vi "rm.server.visualize.get resource entries.vi"(7 "show unmapped?":bool, 8 "error in (no error)":errorcluster, 11 "Item Ref in":T2 format="%.0x") -> (0 "error out":errorcluster, 2 "resource entries":T1[](array[typedef]) {"FPGA CD Ref" format="%.0x"; "reserver" format="%.0x"}, 3 "Item Ref out":T2 format="%.0x")   [LabVIEW 2016, in "RM.Server.lvlib"]
uses:
  RM.Server.lvlib
  <vilib>/NI Veristand/Custom Device API/Custom Device Item Ref.ctl
  viz_entry.ctl
  FPGA-Addon/Source/Shared/FG Action.ctl
  FPGA-Addon/Source/Shared/Constants.vi
  <vilib>/NI Veristand/Custom Device API/Get Item Property (Variant).vi
  <vilib>/NI Veristand/Custom Device API/NI VeriStand - Set Item Property.vi
  <vilib>/NI Veristand/Custom Device API/Set Item Property (Variant).vi
  <vilib>/NI Veristand/Custom Device API/Get Item Property (Dependent Node Pointer).vi
  <vilib>/NI Veristand/Custom Device API/Get Item Property (String).vi
  <vilib>/NI VeriStand/Custom Device API/Custom Device API.lvlib
  FPGA-Addon/Source/Shared/FPGA Addon Shared.lvlib
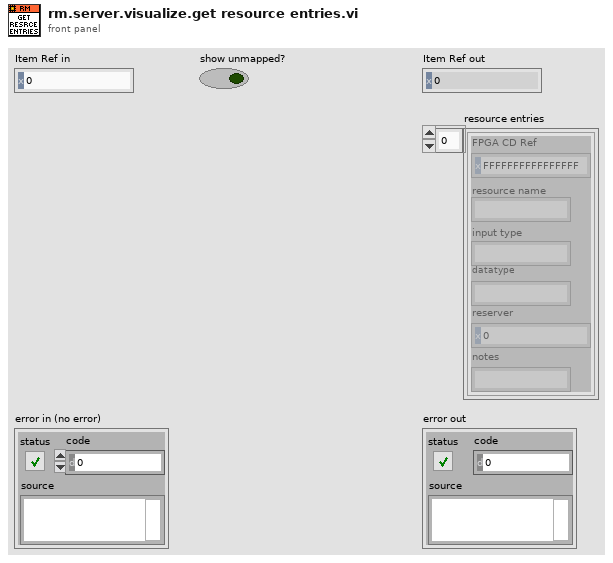
[diagram p1: front panel]
types:
  T1 = typedef "RM.Server.lvlib/viz_entry.ctl" = cluster{"FPGA CD Ref":T2, "resource name":string, "input type":string, "datatype":string, "reserver":T2, "notes":string}
  T2 = typedef "Custom Device API.lvlib/Custom Device Item Ref.ctl" = u64
  T3 = typedef "FPGA Addon Shared.lvlib/FG Action.ctl" = enum8{"GET", "SET"}
  T4 = typedef "Custom Device API.lvlib/Custom Device Item Info.ctl" = cluster{"Name":string, "Is Channel":bool, "GUID":string, "Is Waveform":bool}
  T5 = typedef "FPGA Addon Shared.lvlib/Register Information.ctl" = cluster{"Name":string, "Data Type":T6, "Default Value":variant}
  T6 = typedef "FPGA Addon Shared.lvlib/Data Type.ctl" = enum8{"<Null>", "I8", "I16", "I32", "I64", "U8", "U16", "U32", "U64", "SGL", "Boolean", "Analog PWM In Settings", "Analog PWM In", "Digital PWM In Settings", "Digital PWM In", "Digital PWM Out", "Sine Out", "FXP+/-24.5", "FXP+/-16.5", "FXP+/-32.8", "FXP+/-64.32", "FXP+/-16.7", "FXP+/-20.5"}
  T7 = typedef "Fifo_DMA_Config.ctl" = cluster{"Name":string, "Depth":u32, "Write? (Deprecated:Use Implementation)":bool, "Physical Channel":u32, "Base Address":u32, "Data Width":u32, "Data Type":T8, "FXP Properties":variant, "Write Window Address":u32, "Implementation":T9, "Control Set":u32}
  T8 = typedef "niFpgaDataTypeControl.ctl" = enum32{"Boolean", "I8", "I16", "I32", "I64", "U8", "U16", "U32", "U64", "FXP", "CustomControl", "SGL"}
  T9 = typedef "niFpgaDmaChannelImplementation.ctl" = enum16{"niFpgaTargetToHost", "niFpgaHostToTarget", "niFpgaPeerToPeerWriter", "niFpgaPeerToPeerReader", "niCoreTargetToHost", "niCoreHostToTarget"}
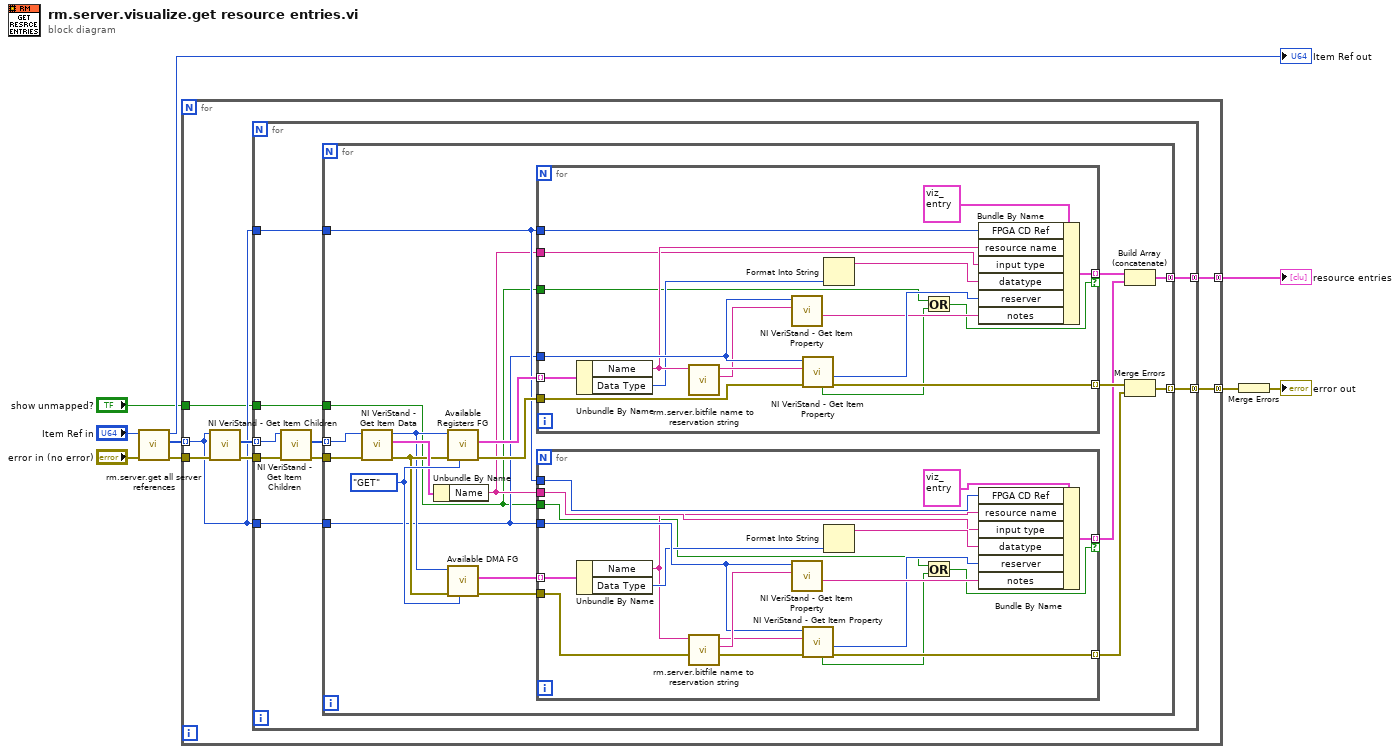
[diagram p0: block diagram]
diagram:
  n1 = call "rm.server.get all server references.vi"("error in (no error)"="error in (no error)", "Item Ref in"="Item Ref in") -> ("error out"=w5:errorcluster, "RM Server refs out"=w6:T2[], "Item Ref out"=→"Item Ref out":T2)  [unwired: 7 in]
  n2 = for {
    tunnel: w5 -> [w16]
    tunnel: w6 -> [w11] mode=indexing
    tunnel: [w13] -> w8 mode=concatenating
    tunnel: [w12] -> w2 mode=concatenating
    tunnel: "show unmapped?" -> [w10]
    n3 = call <vilib>:"NI VeriStand - Get Item Children.vi"("error in (no error)"=w16, "Item Ref in"=w11) -> ("error out"=w15:errorcluster, "Child Refs"=w14:T2[])  [unwired: 6 in, 2 out]
    n4 = for {
      tunnel: w15 -> [w24]
      tunnel: w14 -> [w22] mode=indexing
      tunnel: w11 -> [w21]
      tunnel: [w20] -> w13 mode=concatenating
      tunnel: [w19] -> w12 mode=concatenating
      tunnel: w11 -> [w18]
      tunnel: w10 -> [w17]
      n5 = call <vilib>:"NI VeriStand - Get Item Children.vi"("error in (no error)"=w24, "Item Ref in"=w22) -> ("error out"=w23:errorcluster, "Child Refs"=w25:T2[])  [unwired: 6 in, 2 out]
      n6 = for {
        tunnel: w23 -> [w31]
        tunnel: w25 -> [w34] mode=indexing
        tunnel: w21 -> [w27]
        tunnel: [w39] -> w20 mode=indexing
        tunnel: [w36] -> w19 mode=concatenating
        tunnel: w18 -> [w42]
        tunnel: w17 -> [w26]
        w35 = FG_Action."GET" ("Action")
        n7 = call <vilib>:"NI VeriStand - Get Item Data.vi"("error in (no error)"=w31, "Item Ref in"=w34) -> ("error out"=w30:errorcluster, "Item Info"=w33:T4, "Item Ref out"=w28:T2)  [unwired: 6 in, 1 out]
        n8 = Unbundle By Name(w33) -> ("Name"=w29:string)
        n9 = call "Available Registers FG.vi"("Action"=w35, "error in (no error)"=w30, "Item Ref"=w28) -> ("error out"=w45:errorcluster, "Available Registers"=w44:T5[])  [unwired: 6 in, 1 out]
        n10 = call "Available DMA FG.vi"("Action"=w35, "error in (no error)"=w30, "Item Ref"=w28) -> ("error out"=w32:errorcluster, "Available DMA"=w43:T7[])  [unwired: 6 in, 1 out]
        n11 = for {
          tunnel: w44 -> [w81] mode=indexing
          tunnel: w27 -> [w78]
          tunnel: w45 -> [w80]
          tunnel: [w76] -> w41 mode=indexing
          tunnel: [w70] -> w38 mode=indexing if=w64
          tunnel: w42 -> [w69]
          tunnel: w29 -> [w67]
          tunnel: w26 -> [w66]
          n12 = Unbundle By Name(w81) -> ("Name"=w74:string, "Data Type"=w73:T6)
          n13 = call "rm.server.bitfile name to reservation string.vi"("Name in bitfile"=w74) -> ("Notes String"=w77:string, "Reservation String"=w79:string)  [unwired: 9 in]
          n14 = call-poly <vilib>:"NI VeriStand - Get Item Property.vi"("Property Name"=w77, "Item Ref in"=w78) -> ("Value"=w71:string)  [unwired: 6 in, 3 out]
          n15 = call-poly <vilib>:"NI VeriStand - Get Item Property.vi"("error in (no error)"=w80, "Property Name"=w79, "Item Ref in"=w78) -> ("error out"=w76:errorcluster, "Dependent Node Ref"=w72:T2, "Found"=w65:bool)  [unwired: 5 in, 1 out]
          n16 = Format Into String(w73) -> (resulting string=w68:string)  [unwired: 3 in, 1 out]
          n17 = Or(x=w66, y=w65) -> (x .or. y?=w64:bool)
          n18 = Bundle By Name(cluster=T1 {"FPGA CD Ref"=18446744073709551615, "resource name"="", "input type"="", "datatype"="", "reserver"=18446744073709551615, "notes"=""} ("visualizer entry"), "FPGA CD Ref"=w69, "resource name"=w74, "input type"=w67, "datatype"=w68, "reserver"=w72, "notes"=w71) -> (w70:T1)
        }
        n19 = for {
          tunnel: w43 -> [w58] mode=indexing
          tunnel: w27 -> [w57]
          tunnel: w42 -> [w56]
          tunnel: w32 -> [w55]
          tunnel: [w54] -> w40 mode=indexing
          tunnel: [w51] -> w37 mode=indexing if=w46
          tunnel: w29 -> [w50]
          tunnel: w26 -> [w48]
          n20 = Unbundle By Name(w58) -> ("Name"=w49:string, "Data Type"=w53:T8)
          n21 = call "rm.server.bitfile name to reservation string.vi"("Name in bitfile"=w49) -> ("Notes String"=w60:string, "Reservation String"=w59:string)  [unwired: 9 in]
          n22 = call-poly <vilib>:"NI VeriStand - Get Item Property.vi"("Property Name"=w60, "Item Ref in"=w57) -> ("Value"=w63:string)  [unwired: 6 in, 3 out]
          n23 = call-poly <vilib>:"NI VeriStand - Get Item Property.vi"("error in (no error)"=w55, "Property Name"=w59, "Item Ref in"=w57) -> ("error out"=w54:errorcluster, "Dependent Node Ref"=w62:T2, "Found"=w47:bool)  [unwired: 5 in, 1 out]
          n24 = Format Into String(w53) -> (resulting string=w52:string)  [unwired: 3 in, 1 out]
          n25 = Or(x=w48, y=w47) -> (x .or. y?=w46:bool)
          n26 = Bundle By Name(cluster=T1 {"FPGA CD Ref"=18446744073709551615, "resource name"="", "input type"="", "datatype"="", "reserver"=18446744073709551615, "notes"=""} ("visualizer entry"), "FPGA CD Ref"=w56, "resource name"=w49, "input type"=w50, "datatype"=w52, "reserver"=w62, "notes"=w63) -> (w51:T1)
        }
        n27 = Build Array (concatenate)(w38, w37) -> (w36:T1[])
        n28 = Merge Errors(w41, w40) -> (w39:errorcluster)
      }
    }
  }
  "resource entries" <- w2
  n29 = Merge Errors(w8) -> (→"error out":errorcluster)
